vi "Filter List.set.vi"(10 "filter list":string[](array[string]), 11 "selection_dropdown in":refnum<class "selection_dropdown.lvclass">) -> (3 "selection_dropdown out":refnum<class "selection_dropdown.lvclass">)   [LabVIEW 2024, in "selection_dropdown.lvclass"]
uses:
  selection_dropdown.lvclass
  selection_dropdown.lvclass/selection_dropdown.ctl
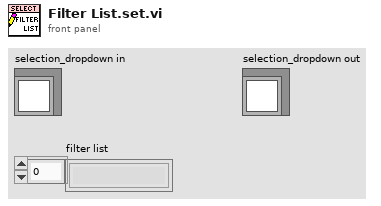
[diagram p1: front panel]
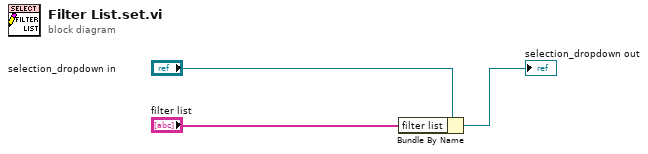
[diagram p0: block diagram]
diagram:
  n1 = Bundle By Name(cluster="selection_dropdown in", "filter list"="filter list") -> (→"selection_dropdown out":refnum<class "selection_dropdown.lvclass">)
